vi "MagnetometerStart.vi"(0 "Device Info":T1={"Serial Number"=-1, "Channel"=0, "Port"=0}, 1 "Data Interval":i32=-1, 2 "Change Trigger":dbl, 11 "error in (no error)":errorcluster, 12 "Connection":u16(ring) items=["No Preference", "Remote", "Local"], 13 "Timeout (mSec)":i32=5000) -> (4 "Phidget ID":u64, 6 "Serial Number Return":i32, 10 "Attached?":bool, 15 "error out":errorcluster)   [LabVIEW 2012, in "Phidget Magnetometer.lvlib"]
doc: "${Magnetometer:StartHeader}"
uses:
  <instrlib>/Phidgets/Phidget Magnetometer/Phidget Magnetometer.lvlib
  <instrlib>/Phidgets/Phidget Common/Phidget Common.lvlib
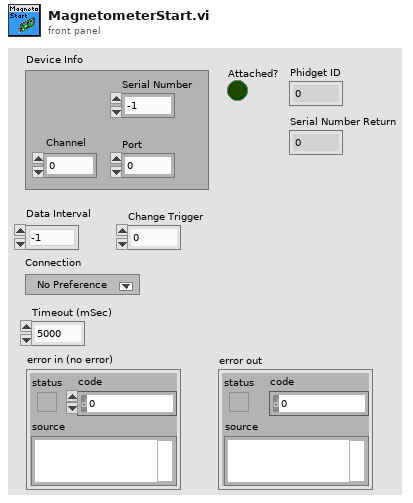
[diagram p1: front panel]
types:
  T1 = cluster{"Serial Number":i32, "Channel":i32, "Port":i32}
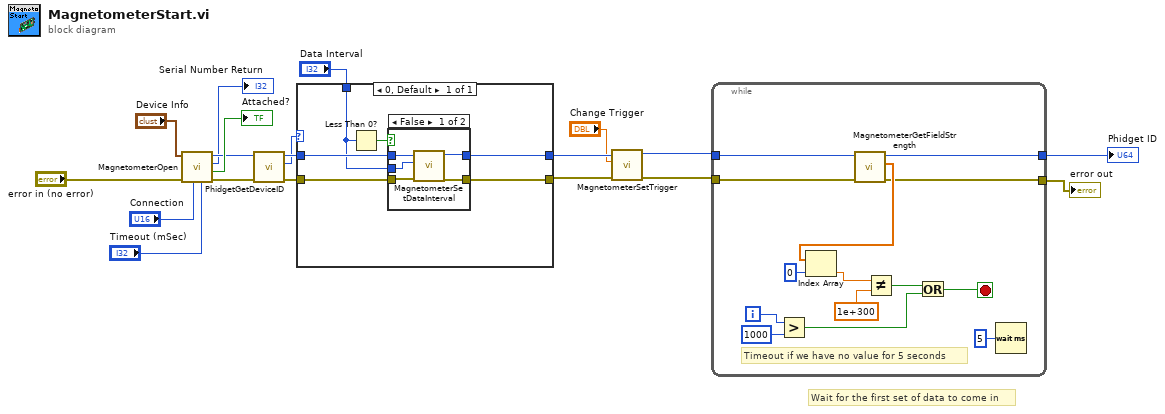
[diagram p0: block diagram]
diagram:
  # "Wait for the first set of data to come in"
  n1 = call <instrlib>:"MagnetometerOpen.vi"("Timeout (mSec)"="Timeout (mSec)", "Connection"="Connection", "error in"="error in (no error)", "Device Info"="Device Info") -> ("error out"=w16:errorcluster, "Attached?"=→"Attached?":bool, "Serial Number Return"=→"Serial Number Return":i32, "Phidget ID"=w15:u64)  [unwired: 4 in]
  n2 = call <instrlib>:"PhidgetGetDeviceID.vi"("error in (no error)"=w16, "Device In"=w15) -> ("error out"=w13:errorcluster, "Devie IDs"=w12:u32, "Device Out"=w14:u64)  [unwired: 6 in]
  n3 = case shown="0, Default" w12 {
    tunnel: w13 -> [w24]
    tunnel: [w20] -> w7
    tunnel: w14 -> [w23]
    tunnel: [w21] -> w6
    tunnel: "Data Interval" -> [w22]
    frame 0, Default {
      n4 = Less Than 0?(x=w22) -> (x < 0?=w25:bool)
      n5 = case shown="False" w25 {
        tunnel: w23 -> [w30 w32]
        tunnel: w24 -> [w29 w31]
        tunnel: [w27 w32] -> w21
        tunnel: [w26 w31] -> w20
        tunnel: w22 -> [w28 _]
        frame False {
          n6 = call <instrlib>:"MagnetometerSetDataInterval.vi"("error in (no error)"=w29, "Interval"=w28, "Device In"=w30) -> ("error out"=w26:errorcluster, "Device Out"=w27:u64)  [unwired: 6 in]
        }
        frame True {
        }
      }
    }
  }
  n7 = call <instrlib>:"MagnetometerSetTrigger.vi"("error in (no error)"=w7, "Change Trigger"="Change Trigger", "Device In"=w6) -> ("error out"=w4:errorcluster, "Device Out"=w5:u64)  [unwired: 6 in]
  n8 = while {
    tunnel: w5 -> [w44]
    tunnel: w4 -> [w43]
    tunnel: [w42] -> w11
    tunnel: [w33] -> w18
    i -> [w40]
    stop <- w38 stop-if-true
    # "Timeout if we have no value for 5 seconds"
    n9 = Greater?(x=w40, y=1000) -> (0:w39:bool)
    n10 = call <instrlib>:"MagnetometerGetFieldStrength.vi"("error in (no error)"=w43, "Device In"=w44) -> ("error out"=w33:errorcluster, "Magneic Field"=w35:dbl[], "Device Out"=w42:u64)  [unwired: 6 in]
    n11 = Index Array(array=w35, index=0) -> (element=w34:dbl)
    n12 = Not Equal?(x=w34, y=1e+300) -> (x != y?=w37:bool)
    n13 = Or(x=w37, y=w39) -> (x .or. y?=w38:bool)
    n14 = Wait (ms)(milliseconds to wait=u32 5) -> ()  [unwired: 1 out]
  }
  "error out" <- w18
  "Phidget ID" <- w11
